vi "testEvaluate.vi"() -> ()   [LabVIEW 2017, in "Transparent Assertions.Tests.lvlib" / "Constraint.lvlib"]
uses:
  Constraint.lvlib
  src/Transparent Assertions/Constraint/Constraint.lvclass
  src/Transparent Assertions/Transparent Assertions.lvlib
panel:
  out "error out":errorcluster
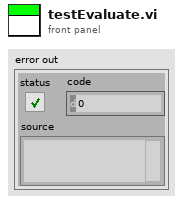
[diagram p1: front panel]
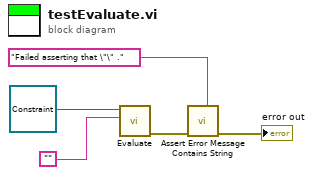
[diagram p0: block diagram]
diagram:
  n1 = call-dynamic "Evaluate.vi"("Actual"="", "Constraint in"=refnum<class "Constraint.lvclass"> refnum ("Constraint.lvlib:Constraint.lvclass")) -> ("error out"=w3:errorcluster)  [unwired: 8 in, 1 out]
  n2 = call "Assert Error Message Contains String.vi"("Expected"="Failed asserting that \"\" .", "error in (no error)"=w3) -> ("error out"=→"error out":errorcluster)  [unwired: 9 in]
